vi "class discovery singleton.vi"(7 "method":T1, 8 "error in":errorcluster, 9 "Folders to Exclude":string[](array[string]), 10 "Plugin Search Paths":path[](array[path]), 11 "Class Name":string) -> (0 "error out":errorcluster, 1 "discovered classes":path[](array[path]), 2 "class path":path, 3 "LabVIEW Object":refnum<class>)   [LabVIEW 2023, in "CEF.lvlib"]
doc: "A functional global variable which provides name-based lookup of classes. When a search path is added, the FGV will locate all classes on disk and use the *filename* to cache them in memory. That is, the class c:\\classes\\foo.lvclass is stored as foo, not as FrameworkClasses.lvlib::Foo.lvclass. The assumption is that anything already in memory can be loaded by other means. When a load is requested, the FGV will first use the name as an input to get lvclass default value by name (which does expect FrameworkClasses.lvlib::Foo.lvclass). Then it will look for foo.lvclass in the list of found classes on disk. Then if all else fails, it will attempt to match a class in memory using a string match.Copyright 2017 National Instruments Corporation\n\nLicensed under the Apache License, Version 2.0 (the \"License\"); you may not use this file except in compliance with the License. You may obtain a copy of the License at http://www.apache.org/licenses/LICENSE-2.0\nUnless required by applicable law or agreed to in writing, software distributed under the License is distributed on an \"AS IS\" BASIS, WITHOUT WARRANTIES OR CONDITIONS OF ANY KIND, either express or implied. See the License for the specific language governing permissions and limitations under the License."
uses:
  CEF.lvlib
  class discovery singleton methods.ctl
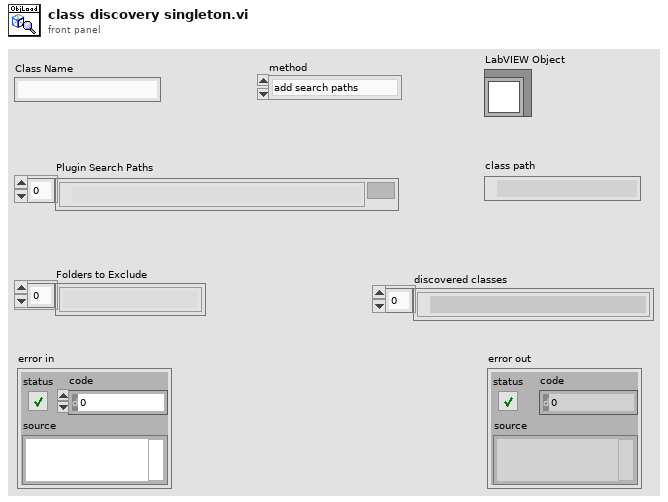
[diagram p1: front panel]
types:
  T1 = typedef "CEF.lvlib/class discovery singleton methods.ctl" = enum16{"add search paths", "load class by name", "list available classes", "get class path", "delete cache"}
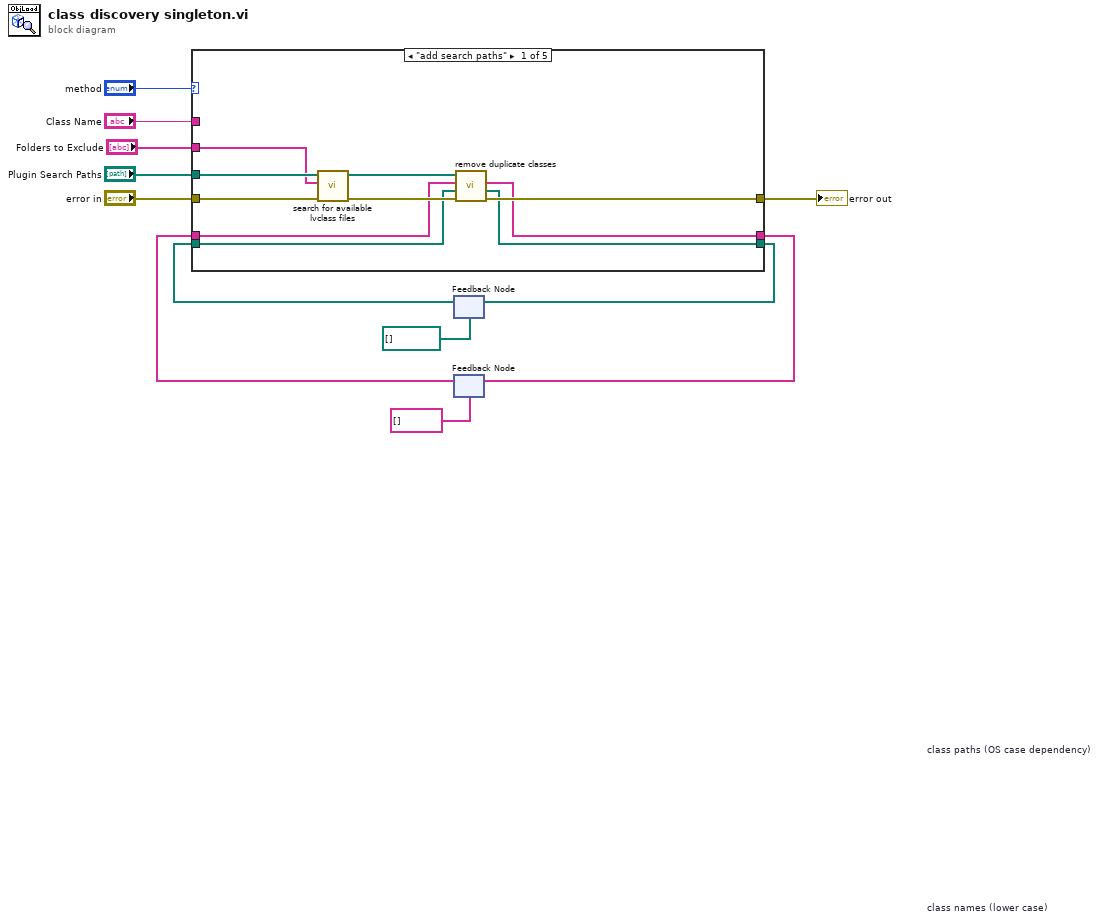
[diagram p0: block diagram]
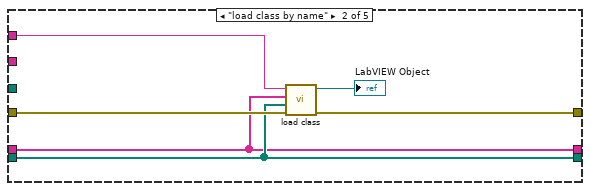
[diagram p2: hidden frame]
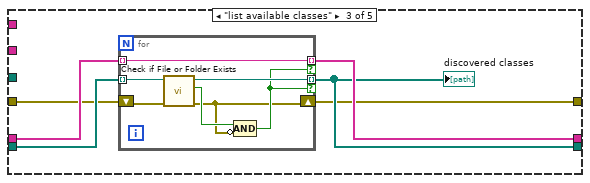
[diagram p3: hidden frame]
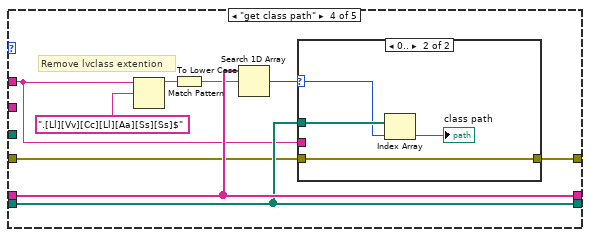
[diagram p4: hidden frame]
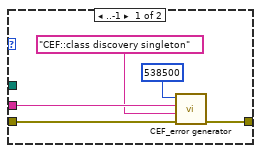
[diagram p5: hidden frame]
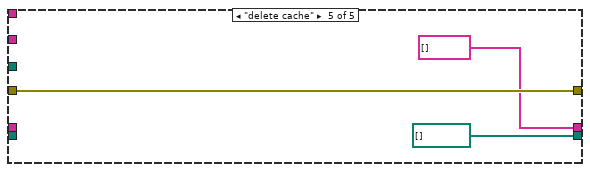
[diagram p6: hidden frame]
diagram:
  n1 = feedback #1 "class paths (OS case dependency)"(path[] [] ("class paths out")) -> (w5:path[])
  n2 = feedback #2 "class names (lower case)"(string[] [] ("class names out")) -> (w7:string[])
  n3 = case shown="\"add search paths\"" "method" {
    tunnel: "error in" -> [w22 w28 w30 w47 w62]
    tunnel: "Plugin Search Paths" -> [w21 _ _ _ _]
    tunnel: [w18 w27 w29 w46 w62] -> w9
    tunnel: w7 -> [w17 w25 w33 w50 _]
    tunnel: [w16 w25 w32 w50 string[] [] ("class names out")] -> w8
    tunnel: [w15 w26 w31 w49 path[] [] ("class paths out")] -> w6
    tunnel: w5 -> [w14 w26 w34 w49 _]
    tunnel: "Class Name" -> [_ w24 _ w44 _]
    tunnel: "Folders to Exclude" -> [w13 _ _ _ _]
    frame "add search paths" {
      n4 = call "search for available lvclass files.vi"("error in"=w22, "Folders to Exclude"=w13, "Plugin Search Paths"=w21) -> ("error out"=w19:errorcluster, "discovered classes"=w20:path[])  [unwired: 7 in]
      n5 = call "remove duplicate classes.vi"("error in"=w19, "class paths in"=w14, "class names in"=w17, "discovered classes"=w20) -> ("error out"=w18:errorcluster, "class paths out"=w15:path[], "class names out"=w16:string[])  [unwired: 5 in]
    }
    frame "load class by name" {
      n6 = call "load class.vi"("error in"=w28, "available class paths"=w26, "available class names"=w25, "Class Name"=w24) -> ("error out"=w27:errorcluster, "Object Out"=→"LabVIEW Object":refnum<class>)  [unwired: 6 in]
    }
    frame "list available classes" {
      n7 = for {
        tunnel: w34 -> [w41] mode=indexing
        tunnel: w33 -> [w39] mode=indexing
        tunnel: [w39] -> w32 mode=indexing if=w37
        tunnel: [w38] -> w31 mode=indexing if=w37
        shift-right: [w35] -> w29
        shift-left: w30 -> [w36]
        n8 = call <vilib>:"Check if File or Folder Exists.vi"("error in (no error)"=w36, "path"=w41) -> ("error out"=w35:errorcluster, "file or folder exists?"=w40:bool, "dup path"=w38:path)  [unwired: 7 in]
        n9 = Compound Arithmetic op=AND(w40, invert w35) -> (w37:bool)
      }
      "discovered classes" <- w31
    }
    frame "get class path" {
      # "Remove lvclass extention"
      n10 = Match Pattern(string=w44, regular expression=".[Ll][Vv][Cc][Ll][Aa][Ss][Ss]$") -> (before substring=w43:string)  [unwired: 1 in, 3 out]
      n11 = To Lower Case(string=w43) -> (all lower case string=w45:string)
      n12 = Search 1D Array(1D array=w50, element=w45) -> (index of element=w48:i32)  [unwired: 1 in]
      n13 = case shown="0.." w48 {
        selector: w48 -> [_ w58]
        tunnel: w49 -> [_ w59]
        tunnel: w47 -> [w54 w57]
        tunnel: [w55 w57] -> w46
        tunnel: w44 -> [w53 _]
        frame ..-1 {
          n14 = call "CEF_error generator.vi"("error in"=w54, "source"="CEF::class discovery singleton", "append error message"=w53, "error code (0)"=538500) -> ("error out"=w55:errorcluster)  [unwired: 5 in]
        }
        frame 0.. {
          n15 = Index Array(array=w59, index=w58) -> (element=→"class path":path)
        }
      }
    }
    frame "delete cache" {
    }
  }
  "error out" <- w9
  n16 = feedback-in #1(w6) -> ()
  n17 = feedback-in #2(w8) -> ()
